vi "Cache_Path Global_Write.vi"(8 "error in (no error)":errorcluster, 11 "Cache Path":path) -> (0 "error out":errorcluster, 1 "Success?":bool, 3 "Non-unique Class Names":string[](array[string]))   [LabVIEW 2019, in "ClassLoader.lvlib"]
uses:
  ClassLoader.lvlib
  <vilib>/Utility/config.llb/NI_LVConfig.lvlib
  Cache_Path Global.vi
  <vilib>/Utility/config.llb/Read Key (String).vi
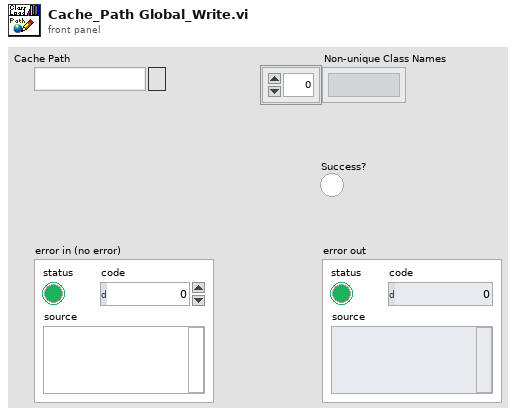
[diagram p1: front panel]
types:
  T1 = typedef "NI_LVConfig.lvlib/Config Data RefNum.ctl" = refnum<k1>
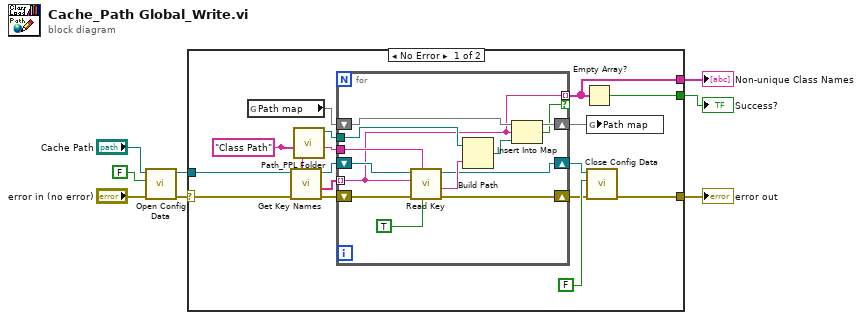
[diagram p0: block diagram]
diagram:
  n1 = call <vilib>:"Open Config Data.vi"("error in (no error)"="error in (no error)", "create file if necessary (T)"=FALSE, "configuration file path"="Cache Path") -> ("error out"=w5:errorcluster, "refnum"=w3:T1)  [unwired: 6 in, 1 out]
  n2 = case shown="No Error" w5 {
    selector: w5 -> [w21 w37]
    tunnel: [w12 w37] -> w4
    tunnel: w3 -> [w22 _]
    tunnel: [w11 _] -> w2
    tunnel: [w10 _] -> w1
    frame No Error {
      w18 = "Class Path" ("section")
      n3 = global read "Cache_Path Global.vi" "Path map"() -> (w16:map{string, path})
      n4 = call <vilib>:"Get Key Names.vi"("section"=w18, "error in (no error)"=w21, "refnum"=w22) -> ("error out"=w15:errorcluster, "key names"=w19:string[], "refnum out"=w20:T1)  [unwired: 5 in, 1 out]
      n5 = call "Path_PPL Folder.vi"() -> ("Data Folder Path"=w17:path)  [unwired: 10 in, 1 out]
      n6 = for {
        tunnel: w19 -> [w26] mode=indexing
        tunnel: w18 -> [w34]
        tunnel: w17 -> [w33]
        shift-right: [w29] -> w9
        shift-left: w16 -> [w30]
        shift-right: [w25] -> w13
        shift-left: w15 -> [w31]
        shift-right: [w24] -> w14
        shift-left: w20 -> [w35]
        tunnel: [w26] -> w11 mode=indexing if=w27
        n7 = call-poly <vilib>:"Read Key.vi"("read raw string? (F)"=TRUE, "section"=w34, "error in (no error)"=w31, "key"=w26, "refnum"=w35) -> ("error out"=w25:errorcluster, "value"=w32:string, "refnum out"=w24:T1)  [unwired: 3 in, 1 out]
        n8 = Build Path(base path=w33, name or relative path=w32) -> (appended path=w28:path)
        n9 = Insert Into Map(map in=w30, key=w26, value=w28) -> (map out=w29:map{string, path}, key already included?=w27:bool)  [unwired: 1 out]
      }
      n10 = Empty Array?(array=w11) -> (empty?=w10:bool)
      n11 = global write "Cache_Path Global.vi" "Path map"(w9) -> ()
      n12 = call <vilib>:"Close Config Data.vi"("error in (no error)"=w13, "write file if changed (T)"=FALSE, "refnum"=w14) -> ("error out"=w12:errorcluster)  [unwired: 7 in, 1 out]
    }
    frame Error {
    }
  }
  "error out" <- w4
  "Non-unique Class Names" <- w2
  "Success?" <- w1
